vi "Get Tuner Info.vi"(8 "error in (no error)":errorcluster, 11 "device handle in":T2) -> (0 "error out":errorcluster, 1 "Gains (dB/10)":i32[](array[numeric]), 2 "Tuner Type":T1, 3 "device handle out":T2, 5 "# Available Gains":i32)   [LabVIEW 2021, in "RTL-SDR.lvlib"]
uses:
  RTL-SDR.lvlib
  Controls/RTLSDR Tuner.ctl
  usr/lib64/librtlsdr.so.0
  Controls/Device Handle.ctl
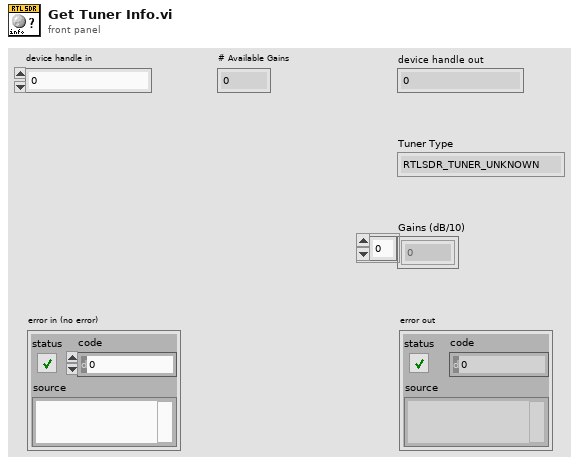
[diagram p1: front panel]
types:
  T1 = typedef "RTL-SDR.lvlib/RTLSDR Tuner.ctl" = enum32{"RTLSDR_TUNER_UNKNOWN", "RTLSDR_TUNER_E4000", "RTLSDR_TUNER_FC0012", "RTLSDR_TUNER_FC0013", "RTLSDR_TUNER_FC2580", "RTLSDR_TUNER_R820T", "RTLSDR_TUNER_R828D"}
  T2 = typedef "RTL-SDR.lvlib/Device Handle.ctl" = u64
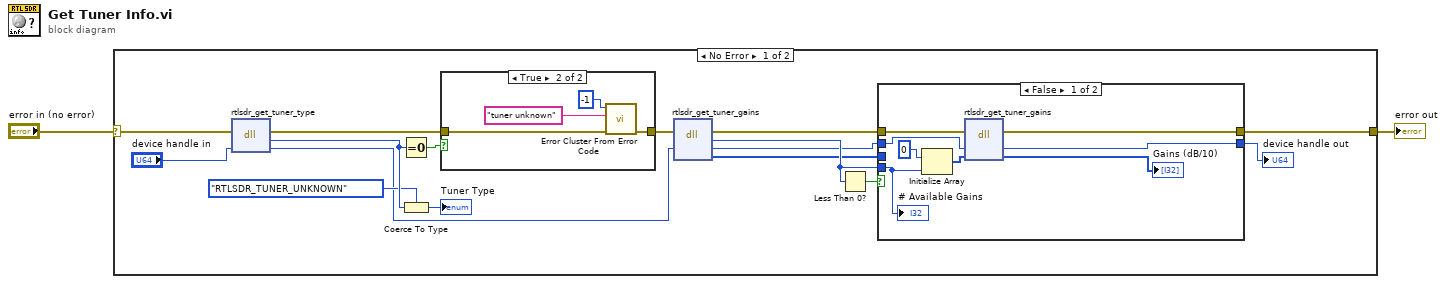
[diagram p0: block diagram]
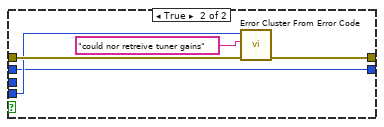
[diagram p2: hidden frame]
diagram:
  n1 = case shown="No Error" "error in (no error)" {
    selector: "error in (no error)" -> [w17 w37]
    tunnel: [w6 w37] -> w2
    frame No Error {
      n2 = dll-call lib="usr/lib64/librtlsdr.so.0" fn="rtlsdr_get_tuner_type"(error in=w17, "dev"="device handle in") -> (error out=w16:errorcluster, "rtlsdr_tuner"=w13:u32, "dev"=w9:u64)  [unwired: 2 in, 1 out]
      n3 = Equal To 0?(x=w13) -> (x = 0?=w15:bool)
      n4 = Coerce To Type(0:w13, 1:RTLSDR_Tuner."RTLSDR_TUNER_UNKNOWN") -> (2:→"Tuner Type":T1)
      n5 = case shown="True" w15 {
        tunnel: w16 -> [w32 w36]
        tunnel: [w32 w35] -> w11
        frame False {
        }
        frame True {
          n6 = call <vilib>:"Error Cluster From Error Code.vi"("error in (no error)"=w36, "error message (\"\")"="tuner unknown" ("error message (\"\")"), "error code (0)"=-1) -> ("error out"=w35:errorcluster)  [unwired: 6 in]
        }
      }
      n7 = dll-call lib="usr/lib64/librtlsdr.so.0" fn="rtlsdr_get_tuner_gains"(error in=w11, "dev"=w9) -> (error out=w10:errorcluster, "return type"=w8:i32, "dev"=w5:u64, "gains"=w3:i32[])  [unwired: 3 in, 1 out]
      n8 = Less Than 0?(x=w8) -> (x < 0?=w7:bool)
      n9 = case shown="False" w7 {
        tunnel: w10 -> [w22 w31]
        tunnel: w8 -> [w26 w30]
        tunnel: [w21 w29] -> w6
        tunnel: w5 -> [w20 w28]
        tunnel: [w19 w28] -> w4
        tunnel: w3 -> [_ _]
        frame False {
          n10 = Initialize Array(0 ("element"), w26) -> (w25:i32[])
          n11 = dll-call lib="usr/lib64/librtlsdr.so.0" fn="rtlsdr_get_tuner_gains"(error in=w22, "dev"=w20, "gains"=w25) -> (error out=w21:errorcluster, "dev"=w19:u64, "gains"=→"Gains (dB/10)":i32[])  [unwired: 3 in, 1 out]
          "# Available Gains" <- w26
        }
        frame True {
          n12 = call <vilib>:"Error Cluster From Error Code.vi"("error in (no error)"=w31, "error message (\"\")"="could nor retreive tuner gains" ("error message (\"\")"), "error code (0)"=w30) -> ("error out"=w29:errorcluster)  [unwired: 6 in]
        }
      }
      "device handle out" <- w4
    }
    frame Error {
    }
  }
  "error out" <- w2
